vi "Test_Highlight_Point_ROI.vi"() -> ()   [LabVIEW 2020]
uses:
  <vilib>/vision/NI_Vision_Development_Module.lvlib
panel:
  in  "Thickness":i32=1 min=1 max=100 step=1
  in  "Draw Overlay":bool
  out "ROI":T1
  in  "stop":bool
  out "Image":T2(plugin-control)
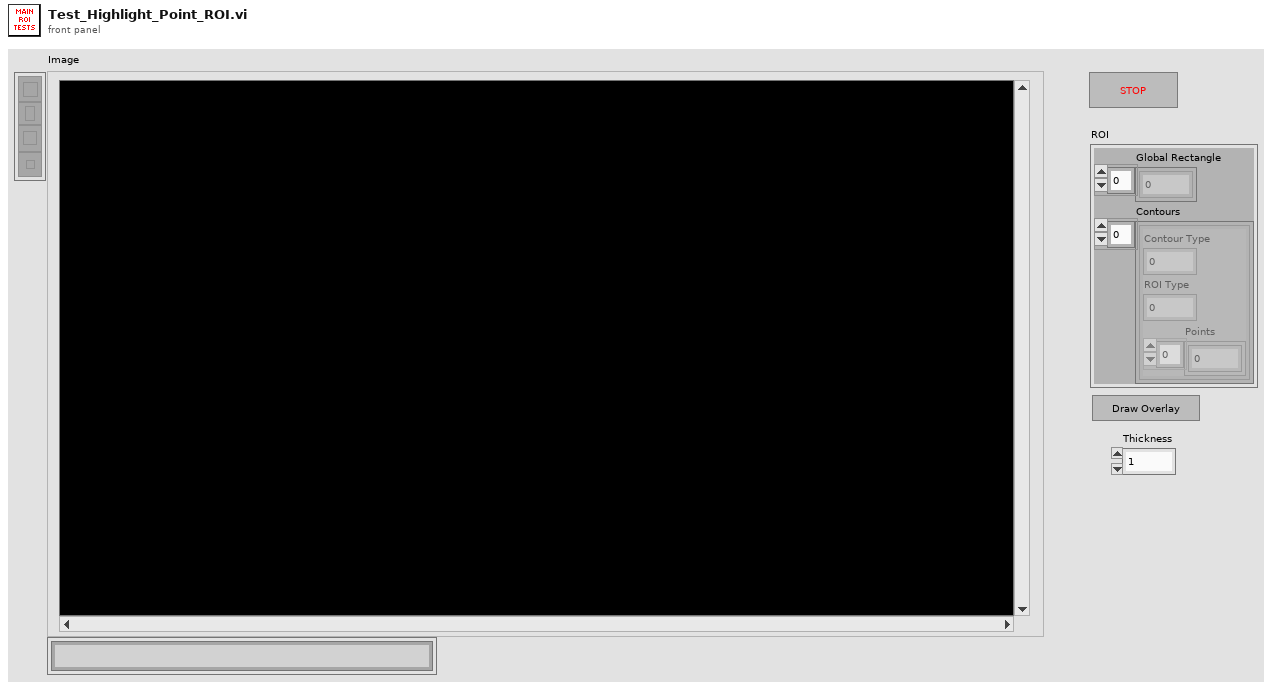
[diagram p1: front panel]
types:
  T1 = cluster{"Global Rectangle":i32[], "Contours":cluster{"Contour Type":u32, "ROI Type":u32, "Points":i32[]}[]}
  T2 = typedef "IMAQ Image.ctl" = refnum<image>
  T3 = typedef "Image Type" = u32
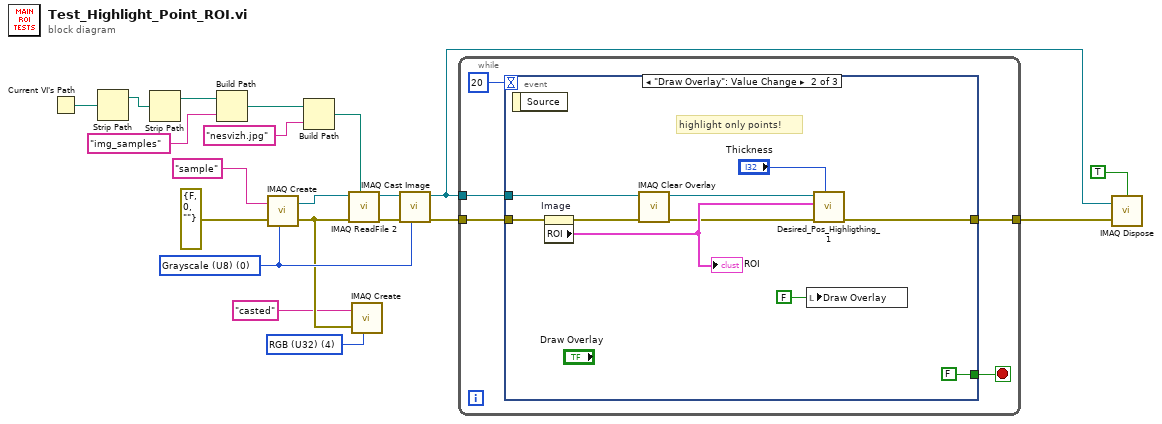
[diagram p0: block diagram]
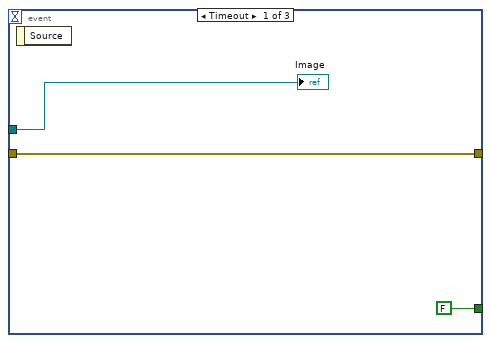
[diagram p2: hidden frame]
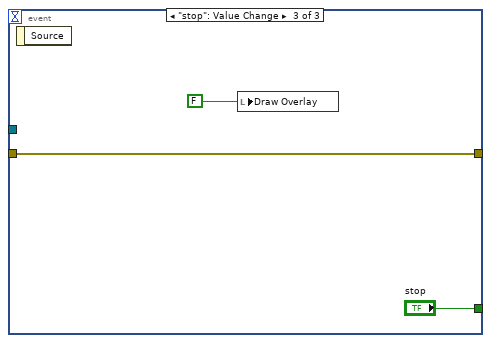
[diagram p3: hidden frame]
diagram:
  w9 = T3 4 items=["Grayscale (U8)", "Grayscale (I16)", "Grayscale (SGL)", "Complex (CSG)", "RGB (U32)", "HSL (U32)", "RGB (U64)", "Grayscale (U16)"] ("Image Type")
  w12 = T3 0 items=["Grayscale (U8)", "Grayscale (I16)", "Grayscale (SGL)", "Complex (CSG)", "RGB (U32)", "HSL (U32)", "RGB (U64)", "Grayscale (U16)"] ("Image Type")
  n1 = Current VI's Path() -> (path=w17:path)
  n2 = Strip Path(path=w17) -> (stripped path=w8:path)  [unwired: 1 out]
  n3 = Strip Path(path=w8) -> (stripped path=w7:path)  [unwired: 1 out]
  n4 = Build Path(base path=w7, name or relative path="img_samples") -> (appended path=w5:path)
  n5 = call "IMAQ Create"("Image Name"="sample", "Image Type"=w12, "error in (no error)"=errorcluster {"status"=FALSE, "code"=0, "source"=""}) -> ("New Image"=w18:T2, "error out"=w11:errorcluster)  [unwired: 2 in]
  n6 = Build Path(base path=w5, name or relative path="nesvizh.jpg") -> (appended path=w15:path)
  n7 = call "IMAQ ReadFile 2"("File Path"=w15, "error in (no error)"=w11, "Image"=w18) -> ("error out"=w14:errorcluster, "Image Out"=w13:T2)  [unwired: 4 in, 3 out]
  n8 = call "IMAQ Create"("Image Name"="casted", "Image Type"=w9, "error in (no error)"=w11) -> ()  [unwired: 2 in, 2 out]
  n9 = call "IMAQ Cast Image"("Image Type"=w12, "error in (no error)"=w14, "Image Src"=w13) -> ("error out"=w4:errorcluster, "Image Dst Out"=w2:T2)  [unwired: 7 in]
  n10 = while {
    tunnel: w4 -> [w24]
    tunnel: w2 -> [w25]
    tunnel: [w22] -> w3
    stop <- w21 stop-if-true
    n11 = event shown="[1] \"Draw Overlay\": Value Change" {
      selector: _ -> [_ _ _]
      dyn-events: _ -> [_ _ _]
      timeout: 20 -> [_ _ _]
      tunnel: w25 -> [w27 w32 _]
      tunnel: w24 -> [w26 w34 w40]
      tunnel: [w26 w35 w40] -> w22
      tunnel: [FALSE ("stop") FALSE ("stop") "stop"] -> w21
      event Timeout {
        n12 = event-data() -> ()  [unwired: 1 in, 1 out]
        "Image" <- w27
      }
      event "Draw Overlay": Value Change {
        # "highlight only points!"
        n13 = event-data() -> ()  [unwired: 1 in, 1 out]
        n14 = property on="Image" class="ImageControl"(error in=w34) -> (error out=w33:errorcluster, "ROI"=w36:T1)  [unwired: 1 in, 1 out]
        "ROI" <- w36
        n15 = call "IMAQ Clear Overlay"("error in (no error)"=w33, "Image"=w32) -> ("error out"=w30:errorcluster, "Image Out"=w31:T2)  [unwired: 8 in]
        n16 = local write "Draw Overlay"(FALSE ("Draw Overlay")) -> ()
        n17 = call "Desired_Pos_Highligthing_1.vi"("[IN] Thickness"="Thickness", "error IN"=w30, "[IN] ROI"=w36, "[IN] Image"=w31) -> ("error OUT"=w35:errorcluster)  [unwired: 7 in]
      }
      event "stop": Value Change {
        n18 = event-data() -> ()  [unwired: 1 in, 1 out]
        n19 = local write "Draw Overlay"(FALSE ("Draw Overlay")) -> ()
      }
    }
  }
  n20 = call "IMAQ Dispose"("All Images? (No)"=TRUE, "Image"=w2, "error in (no error)"=w3) -> ()  [unwired: 3 in, 1 out]
